vi "Get Event Error.vi"(8 "error in (no error)":errorcluster caption="entrée d'erreur (pas d'erreur)", 11 "Class Instrument Log_File en entrée":refnum<class "Class Instrument Log_File.lvclass">) -> (0 "error out":errorcluster caption="sortie d'erreur", 2 "Event Error":refnum<user-event>, 3 "Class Instrument Log_File en sortie":refnum<class "Class Instrument Log_File.lvclass">)   [LabVIEW 2020, in "Library Instrument & Equipement.lvlib" / "Library Instruments.lvlib" / "Class Instrument Log_File.lvclass"]
uses:
  Class Instrument Log_File.lvclass
  Class Instrument Log_File.lvclass/Class Instrument Log_File.ctl
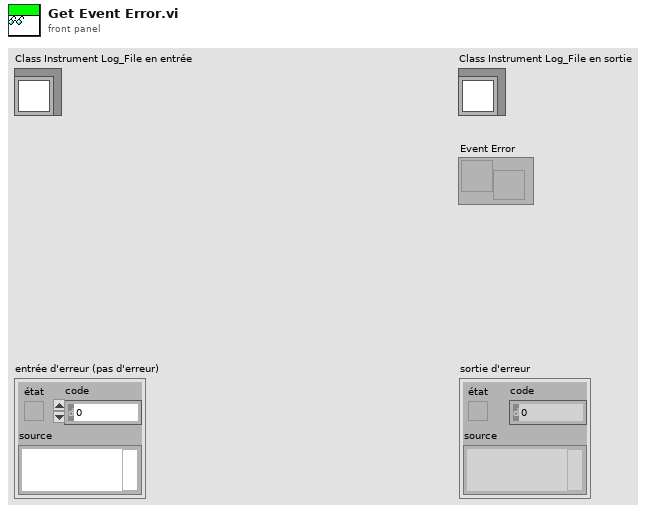
[diagram p1: front panel]
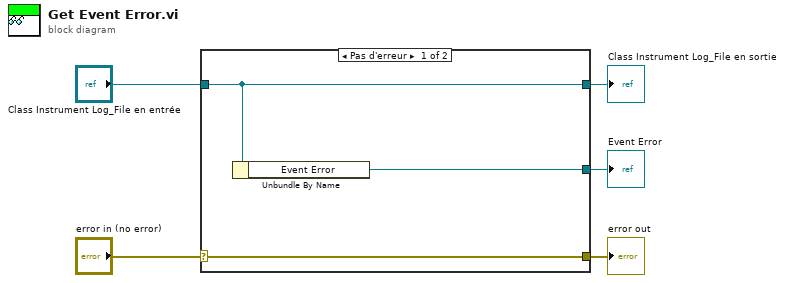
[diagram p0: block diagram]
diagram:
  n1 = case shown="Pas d'erreur" "error in (no error)" {
    selector: "error in (no error)" -> [w8 w9]
    tunnel: [w8 w9] -> w4
    tunnel: [w7 w10] -> w2
    tunnel: "Class Instrument Log_File en entrée" -> [w7 w10]
    tunnel: [w6 _] -> w1
    frame No Error {
      n2 = Unbundle By Name(w7) -> ("Event Error"=w6:refnum<user-event>)
    }
    frame Error {
    }
  }
  "error out" <- w4
  "Class Instrument Log_File en sortie" <- w2
  "Event Error" <- w1
